vi "Fetch Data - PAE.vi"(8 "error in":errorcluster, 10 "Test Configuration":T2={"Expected DUT Gain (dB)"=17.5, "Max Linear Range (dBm)"=-10.0, "Compression Point (dB)"=1.0, "Pout at Pin (dBm)"=1.0, "RFSG Frequency Start (Hz)"=6000000000.0, "RFSG Frequency Stop (Hz)"=18000000000.0, "RFSG Number of Frequency Step"=10, "Power Start (dBm)"=-20.0, "Power Stop(dBm)"=1.0, "Power Step Size (dB)"=4.0, "RBW (Hz)"=5000000.0, "Modes"={"RF Measurement Interval (s)"=0.001, "DC Measurement Interval (s)"=0.0, "Power Stimulus Mode"=enum."Constant Power and RF", "CP_CW_DC Source Delay (s)"=0.0002, "CP_PRF_RF Pulse Width (s)"=0.0009, "CP_PRF_PRI (s)"=0.015, "CP_PRF_DC Source Delay (s)"=0.0, "CP_PRF_RFmx Trigger Delay (s)"=0.2, "PP_PRF_RF Pulse Width (s)"=0.0, "PP_PRF_PRI (s)"=0.0, "PP_PRF_DC Pulse Width (s)"=0.0008, "PP_PRF_Bias Voltage Level (V)"=0.0, "PP_PRF_Bias Current Limit (A)"=0.2, "PP_PRF_DC Source Delay (s)"=0.0, "PP_PRF_RFmx Trigger Delay (s)"=0.0}} {"Pout at Pin (dBm)" format="%#pdBm"; "Modes"."PP_PRF_RFmx Trigger Delay (s)" format="%#ps"; "Modes"."PP_PRF_DC Source Delay (s)" format="%#ps"; "Modes"."PP_PRF_Bias Current Limit (A)" format="%#pA"; "Modes"."PP_PRF_Bias Voltage Level (V)" format="%#pV"; "Modes"."PP_PRF_DC Pulse Width (s)" format="%#ps"; "Modes"."PP_PRF_PRI (s)" format="%#ps"; "Modes"."PP_PRF_RF Pulse Width (s)" format="%#ps"; "Modes"."CP_PRF_RFmx Trigger Delay (s)" format="%#ps"; "Modes"."CP_PRF_DC Source Delay (s)" format="%#ps"; "Modes"."CP_PRF_PRI (s)" format="%#ps"; "Modes"."CP_PRF_RF Pulse Width (s)" format="%#ps"; "Modes"."CP_CW_DC Source Delay (s)" format="%#ps"; "Modes"."DC Measurement Interval (s)" format="%#_6p"; "RFSG Frequency Stop (Hz)" format="%#_6p"; "Power Start (dBm)" format="%#_6p"; "Power Stop(dBm)" format="%#_6p"; "RFSG Frequency Start (Hz)" format="%#_6p"; "Expected DUT Gain (dB)" step=1.0 format="%#_6p"}, 11 "PAE Reference in":T4) -> (0 "error out":errorcluster, 2 "Data":T1, 3 "PAE Reference out":T4)   [LabVIEW 2023]
uses:
  <vilib>/niPAEML/Typedefs/Session Handle.ctl
  <vilib>/niPAEML/PAE Reference.lvclass
  Controls/Test Config - Compression.ctl
  Controls/Results - Compression.ctl
  <vilib>/niPAEML/Fetch PAE (Trace).vi
  <vilib>/niPAEML/PAE Measurement.lvlib
panel:
  out "PAE vs Pin per Freq":T3(graph)
  out "DC Average Power":T3(graph)
  out "Linear Gain vs Freq":cluster{dbl[], dbl[]}(graph)
  out "Pout vs Pin per Freq":T3(graph)
  out "Gain vs Pin per Freq":T3(graph)
  out "OPxdb vs Freq":T5(graph)
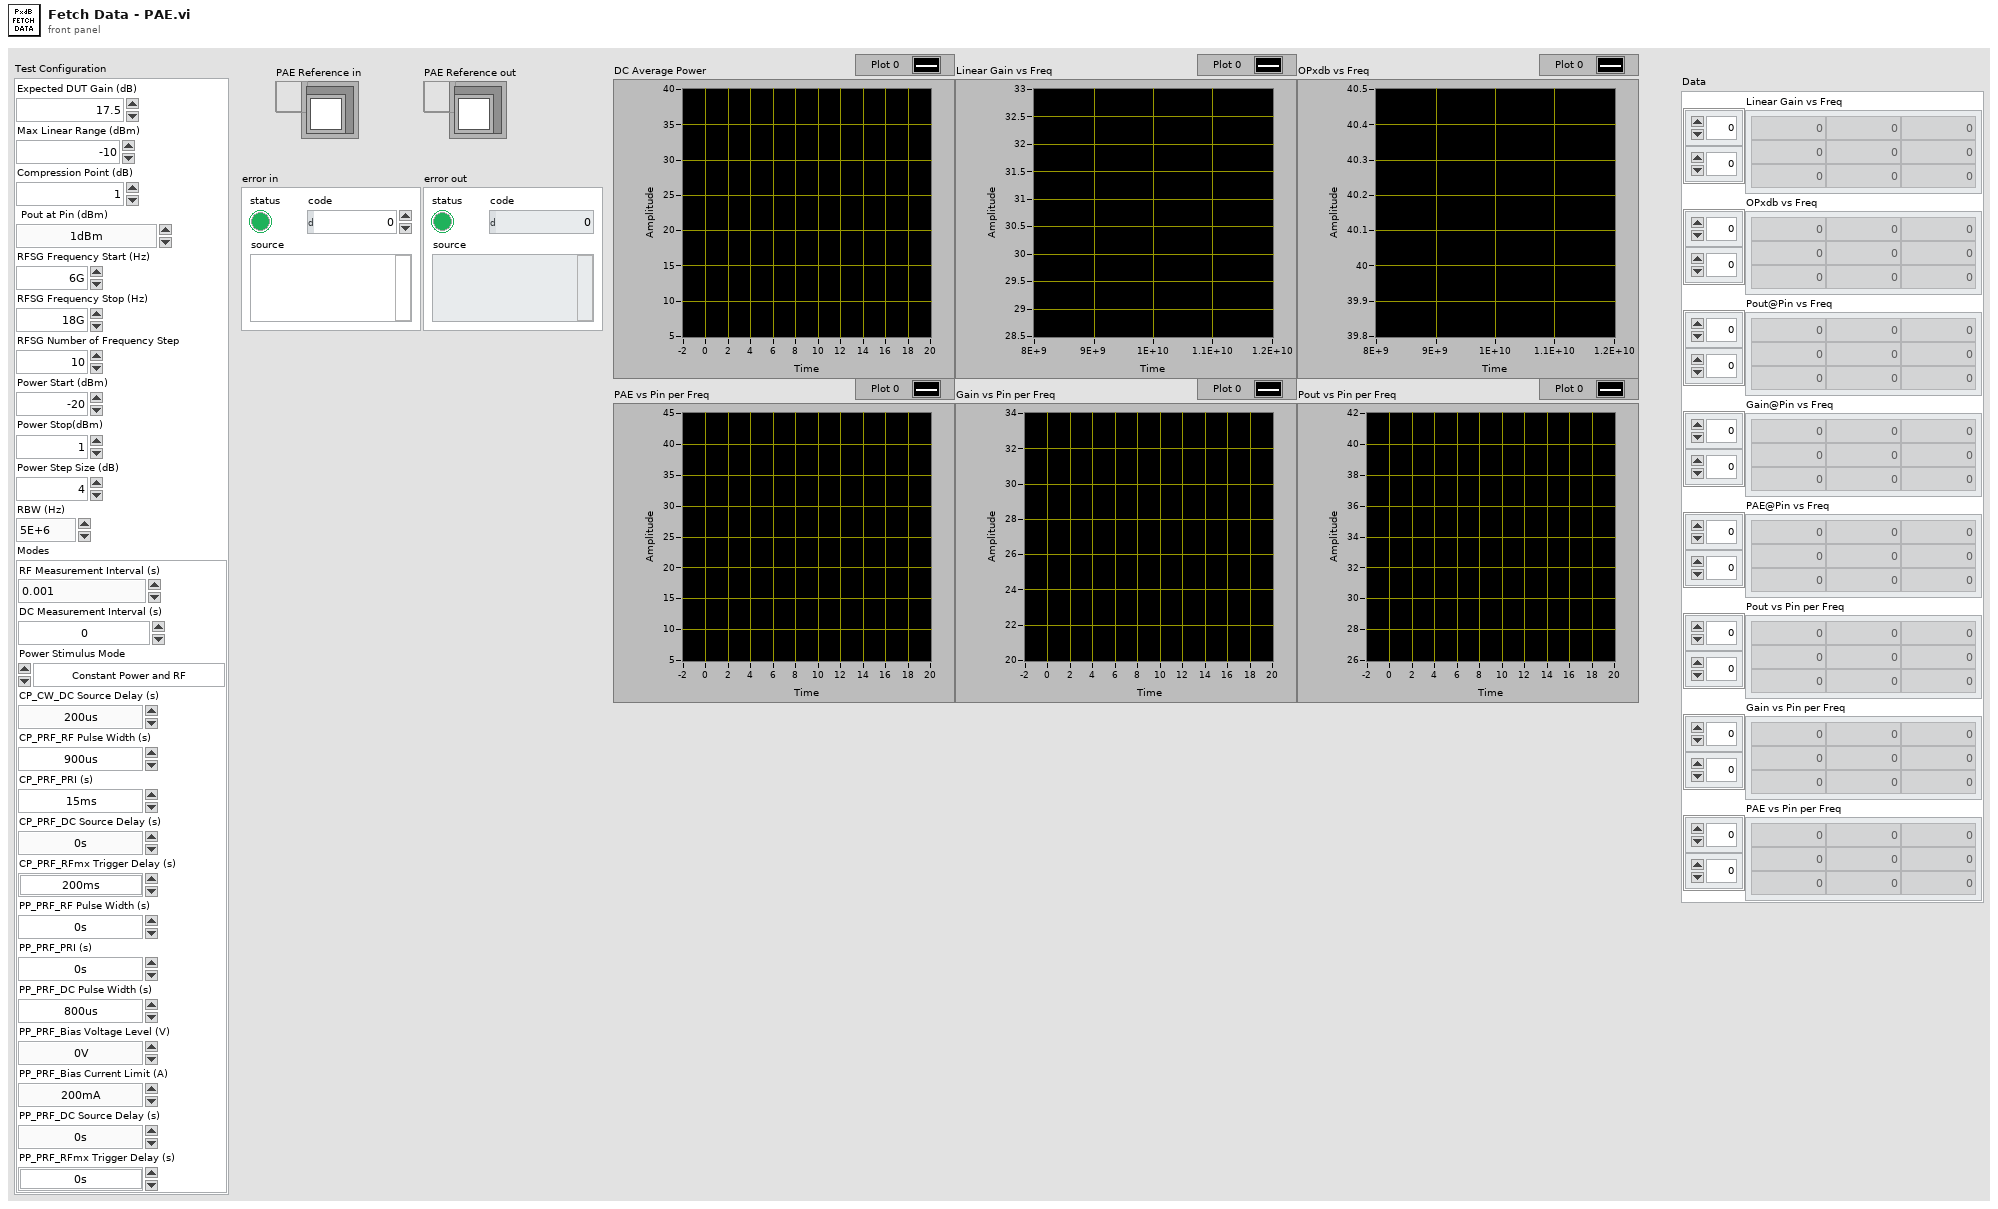
[diagram p1: front panel]
types:
  T1 = typedef "Results - Compression.ctl" = cluster{"Linear Gain vs Freq":dbl[][], "OPxdb vs Freq":dbl[][], "Pout@Pin vs Freq":dbl[][], "Gain@Pin vs Freq":dbl[][], "PAE@Pin vs Freq":dbl[][], "Pout vs Pin per Freq":dbl[][], "Gain vs Pin per Freq":dbl[][], "PAE vs Pin per Freq":dbl[][]}
  T2 = typedef "Test Config - Compression.ctl" = cluster{"Expected DUT Gain (dB)":dbl, "Max Linear Range (dBm)":dbl, "Compression Point (dB)":dbl, "Pout at Pin (dBm)":dbl, "RFSG Frequency Start (Hz)":dbl, "RFSG Frequency Stop (Hz)":dbl, "RFSG Number of Frequency Step":i32, "Power Start (dBm)":dbl, "Power Stop(dBm)":dbl, "Power Step Size (dB)":dbl, "RBW (Hz)":dbl, "Modes":cluster{"RF Measurement Interval (s)":dbl, "DC Measurement Interval (s)":dbl, "Power Stimulus Mode":enum16{"Constant Power and RF", "Constant Power and Pulsed RF", "Pulsed Power and RF"}, "CP_CW_DC Source Delay (s)":dbl, "CP_PRF_RF Pulse Width (s)":dbl, "CP_PRF_PRI (s)":dbl, "CP_PRF_DC Source Delay (s)":dbl, "CP_PRF_RFmx Trigger Delay (s)":dbl, "PP_PRF_RF Pulse Width (s)":dbl, "PP_PRF_PRI (s)":dbl, "PP_PRF_DC Pulse Width (s)":dbl, "PP_PRF_Bias Voltage Level (V)":dbl, "PP_PRF_Bias Current Limit (A)":dbl, "PP_PRF_DC Source Delay (s)":dbl, "PP_PRF_RFmx Trigger Delay (s)":dbl}}
  T3 = cluster{"Input Power (dBm)":dbl[], "Gain (dB)":dbl[]}[]
  T4 = typedef "PAE Measurement.lvlib/PAE Reference.lvclass/Session Handle.ctl" = refnum<data-value>
  T5 = typedef "PAE Measurement.lvlib/Power At PxdB.ctl" = cluster{"Frequencies (Hz)":T6, "Powers (dBm)":T6}
  T6 = typedef "PAE Measurement.lvlib/Double Array.ctl" = dbl[]
  T7 = typedef "PAE Measurement.lvlib/Gain Linear Range.ctl" = cluster{"Frequency Levels (Hz)":dbl, "Gain (Linear Range) (dB)":dbl}
  T8 = typedef "PAE Measurement.lvlib/Gain.ctl" = cluster{"Input Power (dBm)":T6, "Gain (dB)":T6}
  T9 = typedef "PAE Measurement.lvlib/Averaged RF Power.ctl" = cluster{"Input Power (dBm)":T6, "Averaged Power (dBm)":T6}
  T10 = typedef "PAE Measurement.lvlib/Averaged DC Power.ctl" = cluster{"Input Power (dBm)":T6, "Averaged Power (Watt)":T6}
  T11 = typedef "PAE Measurement.lvlib/Power Added Efficiency.ctl" = cluster{"Input Power (dBm)":T6, "PAE":T6}
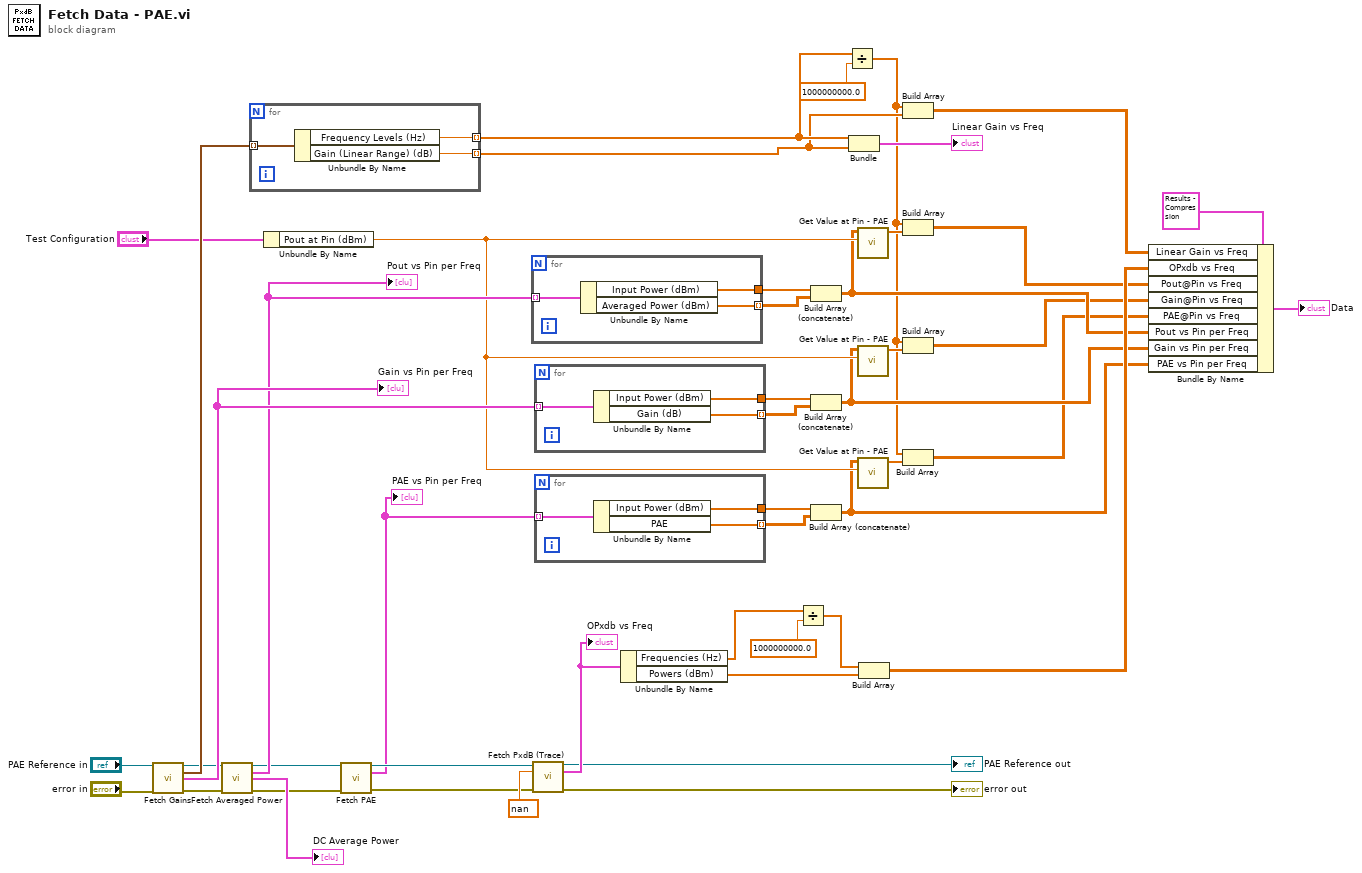
[diagram p0: block diagram]
diagram:
  n1 = call <vilib>:"Fetch Gains.vi"("PAE Reference In"="PAE Reference in", "error in"="error in") -> ("PAE Reference Out"=w31:T4, "Gain (Linear Range) Per Frequency"=w47:T7[], "Gain"=w45:T8[], "error out"=w32:errorcluster)  [unwired: 9 in, 1 out]
  "Gain vs Pin per Freq" <- w45
  n2 = call <vilib>:"Fetch Averaged Power.vi"("PAE Reference In"=w31, "error in"=w32) -> ("PAE Reference Out"=w28:T4, "Averaged RF Power"=w44:T9[], "Averaged DC Power"=→"DC Average Power":T10[], "error out"=w27:errorcluster)  [unwired: 9 in, 1 out]
  "Pout vs Pin per Freq" <- w44
  n3 = for {
    tunnel: w47 -> [w50] mode=indexing
    tunnel: [w49] -> w43 mode=indexing
    tunnel: [w48] -> w42 mode=indexing
    n4 = Unbundle By Name(w50) -> ("Frequency Levels (Hz)"=w49:dbl, "Gain (Linear Range) (dB)"=w48:dbl)
  }
  n5 = Unbundle By Name("Test Configuration") -> ("Pout at Pin (dBm)"=w9:dbl)
  n6 = call-poly <vilib>:"Fetch PAE.vi"("PAE Reference In"=w28, "error in"=w27) -> ("PAE Reference Out"=w26:T4, "Power Added-Efficiency"=w22:T11[], "error out"=w25:errorcluster)  [unwired: 10 in, 1 out]
  "PAE vs Pin per Freq" <- w22
  n7 = for {
    tunnel: w44 -> [w53] mode=indexing
    tunnel: [w52] -> w17
    tunnel: [w51] -> w19 mode=indexing
    n8 = Unbundle By Name(w53) -> ("Input Power (dBm)"=w52:T6, "Averaged Power (dBm)"=w51:T6)
  }
  n9 = call <vilib>:"Fetch PxdB (Trace).vi"("PAE Reference In"=w26, "PxdB Not Found Value"=nan, "error in"=w25) -> ("PAE Reference Out"=→"PAE Reference out":T4, "Power Output at PxdB"=w46:T5, "error out"=→"error out":errorcluster)  [unwired: 8 in, 2 out]
  "OPxdb vs Freq" <- w46
  n10 = for {
    tunnel: w45 -> [w56] mode=indexing
    tunnel: [w55] -> w12
    tunnel: [w54] -> w40 mode=indexing
    n11 = Unbundle By Name(w56) -> ("Input Power (dBm)"=w55:T6, "Gain (dB)"=w54:T6)
  }
  n12 = for {
    tunnel: w22 -> [w59] mode=indexing
    tunnel: [w58] -> w2
    tunnel: [w57] -> w21 mode=indexing
    n13 = Unbundle By Name(w59) -> ("Input Power (dBm)"=w58:T6, "PAE"=w57:T6)
  }
  n14 = Unbundle By Name(w46) -> ("Frequencies (Hz)"=w37:T6, "Powers (dBm)"=w41:T6)
  n15 = Divide(x=w37, y=1000000000.0 ("Frequency Levels (Hz)")) -> (x/y=w36:T6)
  n16 = Build Array (concatenate)(w17, w19) -> (w8:dbl[][])
  n17 = Build Array (concatenate)(w12, w40) -> (w7:dbl[][])
  n18 = Build Array (concatenate)(w2, w21) -> (w6:dbl[][])
  n19 = Divide(x=w43, y=1000000000.0 ("Frequency Levels (Hz)")) -> (x/y=w1:dbl[])
  n20 = Bundle(w43, w42) -> (→"Linear Gain vs Freq":cluster{dbl[], dbl[]})  [unwired: 1 in]
  n21 = call "Get Value at Pin - PAE.vi"("Target Pin (dBm)"=w9, "Measurement"=w8) -> ("Value(s) at Pin"=w18:dbl[])  [unwired: 9 in]
  n22 = call "Get Value at Pin - PAE.vi"("Target Pin (dBm)"=w9, "Measurement"=w7) -> ("Value(s) at Pin"=w13:dbl[])  [unwired: 9 in]
  n23 = call "Get Value at Pin - PAE.vi"("Target Pin (dBm)"=w9, "Measurement"=w6) -> ("Value(s) at Pin"=w16:dbl[])  [unwired: 9 in]
  n24 = Build Array(w36, w41) -> (w10:dbl[][])
  n25 = Build Array(w1, w42) -> (w11:dbl[][])
  n26 = Build Array(w1, w18) -> (w5:dbl[][])
  n27 = Build Array(w1, w13) -> (w4:dbl[][])
  n28 = Build Array(w1, w16) -> (w3:dbl[][])
  n29 = Bundle By Name(cluster=T1 {"Linear Gain vs Freq"=[[8.0], [32.50650691986084]], "OPxdb vs Freq"=[[8.0], [39.831942473969086]], "Pout@Pin vs Freq"=[[-2.0, -1.0, 0.0, 1.0, 2.0, 3.0, 4.0, 5.0, 6.0, 7.0, 8.0, 9.0, 10.0, 11.0, 12.0, 13.0, 14.0, 15.0, 16.0, 17.0, 18.0, 19.0, 20.0], [0.0, 0.0, 0.0, 0.0, 0.0, 0.0, 0.0, 0.0, 0.0, 0.0, 0.0, 0.0, 0.0, 0.0, 0.0, 0.0, 0.0, 0.0, 0.0, 0.0, 0.0, 0.0, 0.0]], "Gain@Pin vs Freq"=[[-2.0, -1.0, 0.0, 1.0, 2.0, 3.0, 4.0, 5.0, 6.0, 7.0, 8.0, 9.0, 10.0, 11.0, 12.0, 13.0, 14.0, 15.0, 16.0, 17.0, 18.0, 19.0, 20.0], [0.0, 0.0, 0.0, 0.0, 0.0, 0.0, 0.0, 0.0, 0.0, 0.0, 0.0, 0.0, 0.0, 0.0, 0.0, 0.0, 0.0, 0.0, 0.0, 0.0, 0.0, 0.0, 0.0]], "PAE@Pin vs Freq"=[[-2.0, -1.0, 0.0, 1.0, 2.0, 3.0, 4.0, 5.0, 6.0, 7.0, 8.0, 9.0, 10.0, 11.0, 12.0, 13.0, 14.0, 15.0, 16.0, 17.0, 18.0, 19.0, 20.0], [0.0, 0.0, 0.0, 0.0, 0.0, 0.0, 0.0, 0.0, 0.0, 0.0, 0.0, 0.0, 0.0, 0.0, 0.0, 0.0, 0.0, 0.0, 0.0, 0.0, 0.0, 0.0, 0.0]], "Pout vs Pin per Freq"=[[-2.0, -1.0, 0.0, 1.0, 2.0, 3.0, 4.0, 5.0, 6.0, 7.0, 8.0, 9.0, 10.0, 11.0, 12.0, 13.0, 14.0, 15.0, 16.0, 17.0, 18.0, 19.0, 20.0], [31.08539581298828, 31.69837188720703, 32.314453125, 32.92780685424805, 33.55664825439453, 34.217926025390625, 34.885520935058594, 35.570068359375, 36.25977325439453, 36.953948974609375, 37.63573455810547, 38.27639389038086, 38.806419372558594, 39.219512939453125, 39.48764419555664, 39.68962097167969, 39.85409927368164, 39.97601318359375, 40.068267822265625, 40.126644134521484, 40.16401672363281, 40.19040298461914, 40.207820892333984]], "Gain vs Pin per Freq"=[[-2.0, -1.0, 0.0, 1.0, 2.0, 3.0, 4.0, 5.0, 6.0, 7.0, 8.0, 9.0, 10.0, 11.0, 12.0, 13.0, 14.0, 15.0, 16.0, 17.0, 18.0, 19.0, 20.0], [33.08539581298828, 32.69837188720703, 32.314453125, 31.927806854248047, 31.55664825439453, 31.217926025390625, 30.885520935058594, 30.570068359375, 30.25977325439453, 29.953948974609375, 29.63573455810547, 29.27639389038086, 28.806419372558594, 28.219512939453125, 27.48764419555664, 26.689620971679688, 25.85409927368164, 24.97601318359375, 24.068267822265625, 23.126644134521484, 22.164016723632812, 21.19040298461914, 20.207820892333984]], "PAE vs Pin per Freq"=[[-2.0, -1.0, 0.0, 1.0, 2.0, 3.0, 4.0, 5.0, 6.0, 7.0, 8.0, 9.0, 10.0, 11.0, 12.0, 13.0, 14.0, 15.0, 16.0, 17.0, 18.0, 19.0, 20.0], [16.022175326980076, 17.330279638793126, 18.715827631120106, 20.15184442982115, 21.709156454144168, 23.45328567860527, 25.332286684465704, 27.37644162362018, 29.550981736945918, 31.853546109742208, 34.23860687033108, 36.57525607103022, 38.4650452490202, 39.905337010912746, 40.697742059393676, 41.12812961396368, 41.39763236661194, 41.40160485000388, 41.283220944492044, 41.09183607984706, 40.8877654308274, 40.66426219876533, 40.43394630315993]]} ("Data"), "Linear Gain vs Freq"=w11, "OPxdb vs Freq"=w10, "Pout@Pin vs Freq"=w5, "Gain@Pin vs Freq"=w4, "PAE@Pin vs Freq"=w3, "Pout vs Pin per Freq"=w8, "Gain vs Pin per Freq"=w7, "PAE vs Pin per Freq"=w6) -> (→"Data":T1)
